vi "ForwardorBackward.vi"(0 "BoatX":i32, 1 "BoatY":i32, 2 "WaypointX":i32, 3 "Waypoint Y":i32, 4 "Heading \n(Degrees)":i32) -> (5 "In Front (on) \n         /\n Behind (off)":bool)   [LabVIEW 2012]
panel:
  out "x-y":dbl
  out "Angle between\nboat and waypoint":dbl
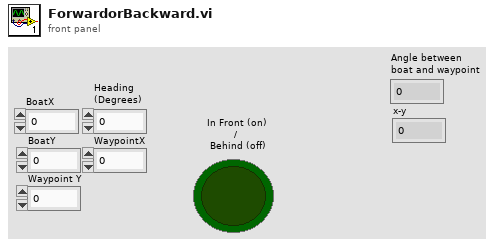
[diagram p1: front panel]
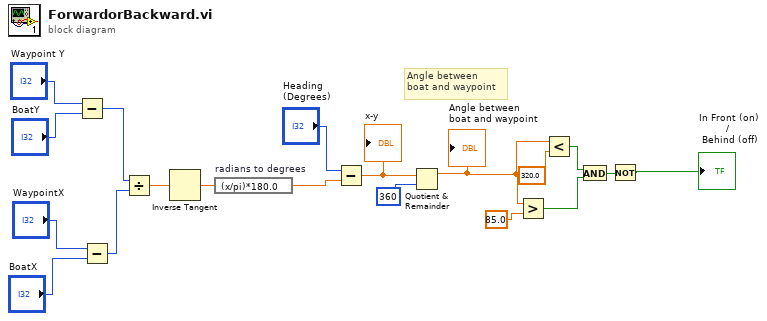
[diagram p0: block diagram]
diagram:
  # "Angle between \nboat and waypoint"
  n1 = Subtract(x="Waypoint Y", y="BoatY") -> (x-y=w19:i32)
  n2 = Subtract(x="WaypointX", y="BoatX") -> (x-y=w18:i32)
  n3 = Divide(x=w19, y=w18) -> (x/y=w17:dbl)
  n4 = Inverse Tangent(1:w17) -> (0:w16:dbl)
  n5 = expression code="(x/pi)*180.0" "radians to degrees"(w16) -> (w14:dbl)
  n6 = Subtract(x="Heading \n(Degrees)", y=w14) -> (x-y=w9:dbl)
  "x-y" <- w9
  n7 = Quotient & Remainder(x=w9, y=360) -> (x-y*floor(x/y)=w6:dbl)  [unwired: 1 out]
  "Angle between\nboat and waypoint" <- w6
  n8 = Greater?(x=w6, y=85.0) -> (0:w3:bool)
  n9 = Less?(x=w6, y=320.0) -> (x < y?=w4:bool)
  n10 = And(x=w4, y=w3) -> (x .and. y?=w2:bool)
  n11 = Not(x=w2) -> (.not. x?=→"In Front (on) \n         /\n Behind (off)":bool)
